vi "Write Value to Signal.vi"(8 "error in (no error)":errorcluster, 10 "Waveform Graph":dynamicdata(graph), 11 "Abstract Sensor in":refnum<class "Abstract Sensor.lvclass">) -> (0 "error out":errorcluster, 3 "Abstract Sensor out":refnum<class "Abstract Sensor.lvclass">)   [LabVIEW 2014, in "Abstract Sensor.lvlib" / "Abstract Sensor.lvclass"]
uses:
  Abstract Sensor.lvclass
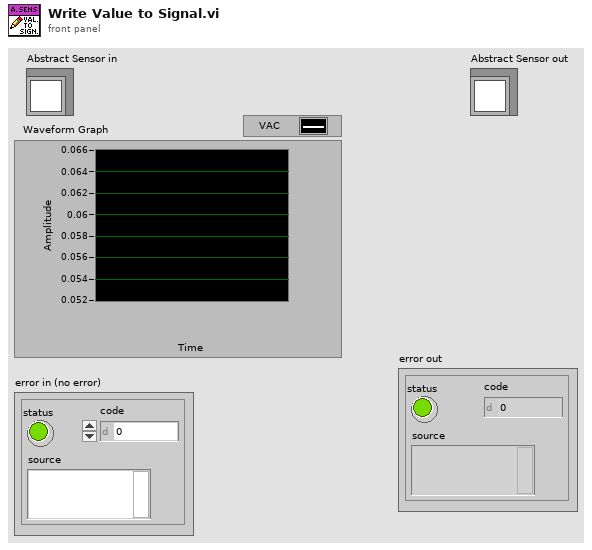
[diagram p1: front panel]
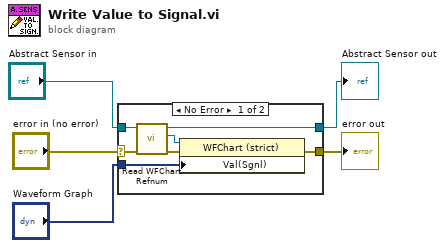
[diagram p0: block diagram]
diagram:
  n1 = case shown="No Error" "error in (no error)" {
    selector: "error in (no error)" -> [w10 w14]
    tunnel: [w7 w14] -> w4
    tunnel: [w11 w13] -> w2
    tunnel: "Abstract Sensor in" -> [w12 w13]
    tunnel: "Waveform Graph" -> [w6 _]
    frame No Error {
      n2 = call-dynamic "Read WFChart Refnum.vi"("error in (no error)"=w10, "Abstract Sensor in"=w12) -> ("error out"=w8:errorcluster, "WFChart Refnum"=w9:refnum<vi>, "Abstract Sensor out"=w11:refnum<class "Abstract Sensor.lvclass">)  [unwired: 7 in]
      n3 = property class="WFChart (strict)"(reference=w9, error in=w8, "Val(Sgnl)"=w6) -> (error out=w7:errorcluster)  [unwired: 1 out]
    }
    frame Error {
    }
  }
  "error out" <- w4
  "Abstract Sensor out" <- w2
